vi "P4CMD File Properties.vi"(8 "error in (no error)":errorcluster, 10 "filename":path, 11 "source control reference in":T1) -> (0 "error out":errorcluster, 2 "status message":string, 3 "source control reference out":T1, 5 "file changed?":bool)   [LabVIEW 2017, in "NI_SCC_P4CMD.lvlib"]
uses:
  <vilib>/SourceControl/Providers/P4CMD/NI_SCC_P4CMD.lvlib
  <vilib>/SourceControl/sccapi/SCCAPI Refnum.ctl
  <vilib>/SourceControl/Providers/P4CMD/P4CMD Mgr Functions.ctl
  <vilib>/SourceControl/Providers/P4CMD/P4CMD Operations.ctl
  <vilib>/SourceControl/support/SCCSup Message Strings GLBL.vi
  <vilib>/SourceControl/sccapi/NI_SCC.lvlib
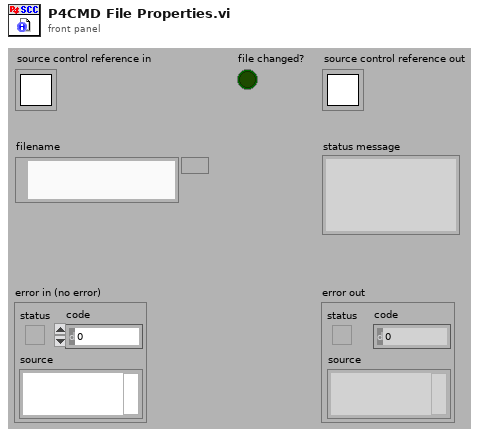
[diagram p1: front panel]
types:
  T1 = typedef "NI_SCC.lvlib/SCCAPI Refnum.ctl" = refnum<k1>
  T2 = typedef "NI_SCC_P4CMD.lvlib/P4CMD Mgr Functions.ctl" = enum16{"Init", "Open", "Set Config Opts", "Initialized?", "IsRefValid?", "Get Config Opts", "Get Global Commands", "Close", "Uninit"}
  T3 = typedef "NI_SCC_P4CMD.lvlib/P4CMD Operations.ctl" = enum16{"get all clients", "get all users", "describe changelist", "sync from depot", "open for edit", "submit to depot", "revert", "add to depot", "remove from depot", "print files revisions", "compare client file", "print depot file contents", "list opened files", "get file info", "lock files", "edit changelist spec", "info", "set variables"}
  T4 = typedef "NI_SCC_P4CMD.lvlib/P4CMD SCC File Status.ctl" = cluster{"source controlled":bool, "open by user":bool, "open by other":bool, "out of date":bool, "deleted":bool, "locked by user":bool, "locked by other":bool, "open for add by user":bool, "open for delete by user":bool}
  T5 = typedef "NI_SCC_P4CMD.lvlib/P4CMD Advanced Options.ctl" = cluster{"lock files?":bool, "suppress dialogs?":bool}
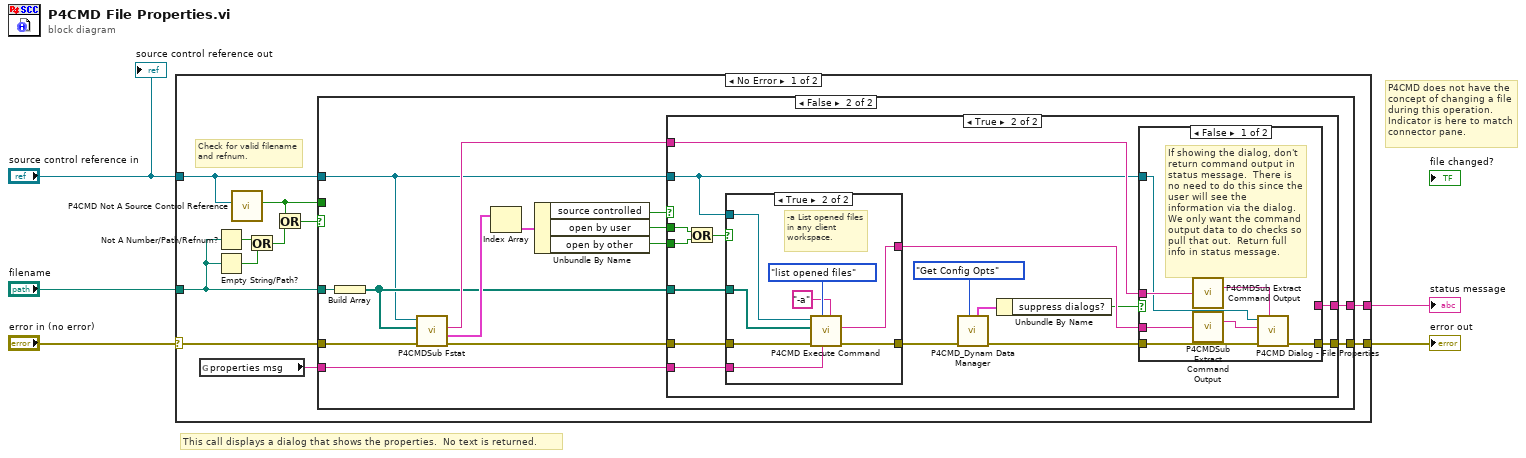
[diagram p0: block diagram]
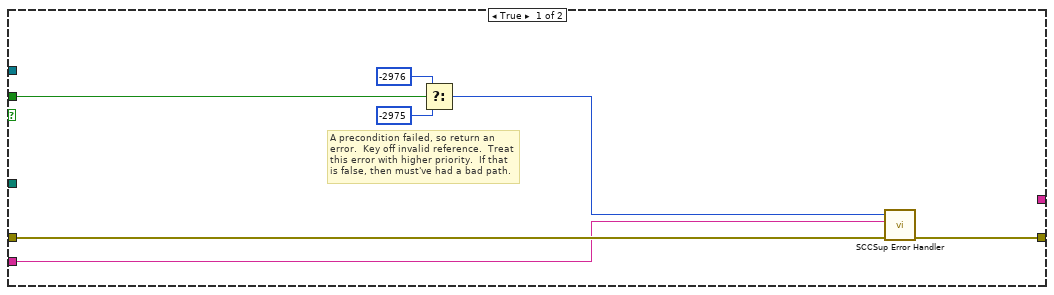
[diagram p2: hidden frame]
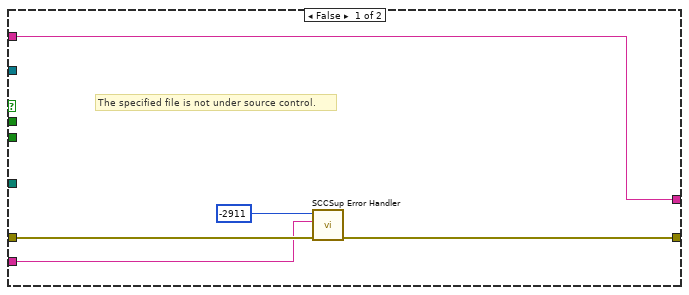
[diagram p3: hidden frame]
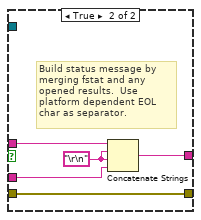
[diagram p4: hidden frame]
diagram:
  # "P4CMD does not have the concept of changing a file during this operation.  Indicator is here to match connector pane."
  # "This call displays a dialog that shows the properties.  No text is returned."
  n1 = case shown="No Error" "error in (no error)" {
    selector: "error in (no error)" -> [w10 w80]
    tunnel: [w8 w80] -> w4
    tunnel: "source control reference in" -> [w13 _]
    tunnel: [w6 _] -> w2
    tunnel: "filename" -> [w9 _]
    frame No Error {
      # "Check for valid filename and refnum."
      n2 = global read "SCCSup Message Strings GLBL.vi" "properties msg"() -> (w7:string)
      n3 = Not A Number/Path/Refnum?(number/path/refnum=w9) -> (NaN/Path/Refnum?=w14:bool)
      n4 = Empty String/Path?(string/path=w9) -> (empty?=w15:bool)
      n5 = call <vilib>:"P4CMD Not A Source Control Reference.vi"("source control reference in"=w13) -> ("not a source control reference?"=w11:bool)  [unwired: 9 in, 1 out]
      n6 = Or(x=w14, y=w15) -> (x .or. y?=w16:bool)
      n7 = Or(x=w11, y=w16) -> (x .or. y?=w12:bool)
      n8 = case shown="False" w12 {
        tunnel: w13 -> [_ w26]
        tunnel: w11 -> [w21 _]
        tunnel: w10 -> [w20 w32]
        tunnel: w9 -> [_ w29]
        tunnel: [w19 w28] -> w8
        tunnel: w7 -> [w17 w25]
        tunnel: [_ w24] -> w6
        frame True {
          # "A precondition failed, so return an error.  Key off invalid reference.  Treat this error with higher priority.  If that is false, then must've had a bad path."
          n9 = Select(t=-2976 ("result"), s=w21, f=-2975 ("result")) -> (s? t:f=w18:i32)
          n10 = call <vilib>:"SCCSup Error Handler.vi"("error in (no error)"=w20, "operation message"=w17, "scc error code"=w18) -> ("error out"=w19:errorcluster)  [unwired: 8 in]
        }
        frame False {
          n11 = Build Array(w29) -> (w27:path[])
          n12 = call <vilib>:"P4CMDSub Fstat.vi"("error in (no error)"=w32, "files"=w27, "source control reference in"=w26) -> ("error out"=w31:errorcluster, "files status"=w36:T4[], "fstat output"=w30:string)  [unwired: 5 in, 1 out]
          n13 = Index Array(array=w36) -> (element=w37:T4)  [unwired: 1 in]
          n14 = Unbundle By Name(w37) -> ("source controlled"=w35:bool, "open by user"=w34:bool, "open by other"=w33:bool)
          n15 = case shown="True" w35 {
            tunnel: w34 -> [_ w56]
            tunnel: w33 -> [_ w55]
            tunnel: w27 -> [_ w54]
            tunnel: w31 -> [w42 w57]
            tunnel: w30 -> [w38 w51]
            tunnel: w26 -> [_ w43]
            tunnel: [w41 w53] -> w28
            tunnel: w25 -> [w39 w52]
            tunnel: [w38 w44] -> w24
            frame False {
              # "The specified file is not under source control."
              n16 = call <vilib>:"SCCSup Error Handler.vi"("error in (no error)"=w42, "operation message"=w39, "scc error code"=-2911 ("error code")) -> ("error out"=w41:errorcluster)  [unwired: 8 in]
            }
            frame True {
              n17 = Or(x=w56, y=w55) -> (x .or. y?=w58:bool)
              n18 = case shown="True" w58 {
                tunnel: [_ w75] -> w50
                tunnel: [w71 w76] -> w47
                tunnel: w57 -> [w71 w77]
                tunnel: w54 -> [_ w78]
                tunnel: w43 -> [_ w74]
                tunnel: w52 -> [_ w73]
                frame False {
                }
                frame True {
                  # "-a List opened files in any client workspace."
                  n19 = call <vilib>:"P4CMD Execute Command.vi"("optional operation parameters"="-a", "operation message"=w73, "p4 operation"=P4CMD_Operations."list opened files", "error in (no error)"=w77, "files"=w78, "source control reference in"=w74) -> ("error out"=w76:errorcluster, "command information"=w75:string)  [unwired: 3 in, 1 out]
                }
              }
              n20 = call <vilib>:"P4CMD_Dynam Data Manager.vi"("function"=P4CMD_Mgr_Functions."Get Config Opts", "error in (no error)"=w47) -> ("error out"=w46:errorcluster, "adv cfg options out"=w48:T5)  [unwired: 4 in, 4 out]
              n21 = Unbundle By Name(w48) -> ("suppress dialogs?"=w45:bool)
              n22 = case shown="False" w45 {
                tunnel: [w65 w70] -> w53
                tunnel: w51 -> [w62 w69]
                tunnel: w50 -> [w63 w66]
                tunnel: w46 -> [w64 w70]
                tunnel: [_ w67] -> w44
                tunnel: w43 -> [w59 _]
                frame False {
                  # "If showing the dialog, don't return command output in status message.  There is no need to do this since the user will see the information via the dialog.\nWe only want the command output data to do checks so pull that out.  Return full info in status message."
                  n23 = call <vilib>:"P4CMDSub Extract Command Output.vi"("bundled message"=w62) -> ("command output"=w61:string)  [unwired: 13 in, 1 out]
                  n24 = call <vilib>:"P4CMDSub Extract Command Output.vi"("bundled message"=w63) -> ("command output"=w60:string)  [unwired: 13 in, 1 out]
                  n25 = call <vilib>:"P4CMD Dialog - File Properties.vi"("fstat data"=w61, "error in (no error)"=w64, "opened data"=w60, "source control reference in"=w59) -> ("error out"=w65:errorcluster)  [unwired: 7 in]
                }
                frame True {
                  w68 = "\r\n"
                  # "Build status message by merging fstat and any opened results.  Use platform dependent EOL char as separator."
                  n26 = Concatenate Strings(w69, w68, w68, w66) -> (w67:string)
                }
              }
            }
          }
        }
      }
    }
    frame Error {
    }
  }
  "error out" <- w4
  "status message" <- w2
  "source control reference out" <- "source control reference in"
